vi "Do Attacked Teams Array.vi"(7 "Teams In":refnum<class "Team.lvclass">[](array[class]), 8 "Team":i32, 10 "Attackers":i32[](array[numeric]), 11 "Square":refnum<class "Square.lvclass">) -> (5 "Teams out":refnum<class "Team.lvclass">[](array[class]))   [LabVIEW 2020, in "SquareBattle.lvlib" / "Square.lvclass"]
uses:
  Square.lvclass
  Square.lvclass/Square.ctl
  Team/Team.lvclass
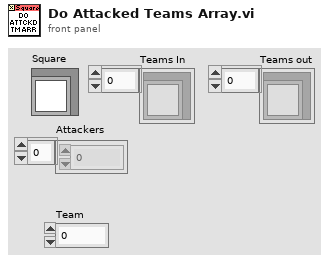
[diagram p1: front panel]
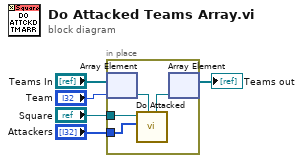
[diagram p0: block diagram]
diagram:
  n1 = in-place {
    in-place-border: "Square" -> [w8]
    in-place-border: "Attackers" -> [w7]
    n2 = in-place-array #1("Teams In", "Team") -> (w9:refnum<class "Team.lvclass">)
    n3 = call "Do Attacked.vi"("Team In"=w9, "Attackers"=w7, "Square"=w8) -> ("Team out"=w6:refnum<class "Team.lvclass">)  [unwired: 8 in]
    n4 = in-place-array #1(w6) -> (→"Teams out":refnum<class "Team.lvclass">[])  [unwired: 1 out]
  }
